vi "PV Software Active BIN Number.vi"(11 "HEX Data (U8)":u8[](array[numeric])) -> (3 "BIN String":string[](array[string]))   [LabVIEW 2023]
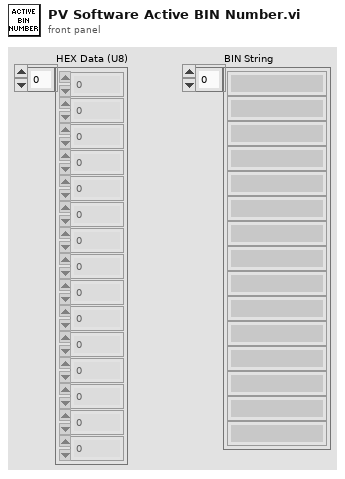
[diagram p1: front panel]
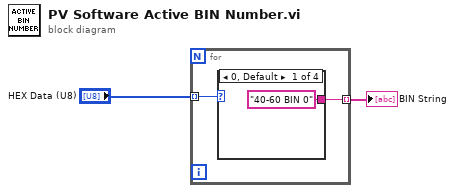
[diagram p0: block diagram]
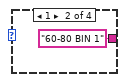
[diagram p2: hidden frame]
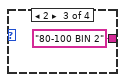
[diagram p3: hidden frame]
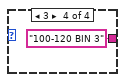
[diagram p4: hidden frame]
diagram:
  n1 = for {
    tunnel: "HEX Data (U8)" -> [w4] mode=indexing
    tunnel: [w3] -> w1 mode=indexing
    n2 = case shown="0, Default" w4 {
      tunnel: ["40-60 BIN 0" "60-80 BIN 1" "80-100 BIN 2" "100-120 BIN 3"] -> w3
      frame 0, Default {
      }
      frame 1 {
      }
      frame 2 {
      }
      frame 3 {
      }
    }
  }
  "BIN String" <- w1
